vi "Poly_Text_Read.vi"(6 "Auto Increment":bool, 8 "error in":errorcluster, 9 "access (0:read/write)":enum16{"read/write", "read-only", "write-only"}(ring), 10 "operation (0:open)":T1(ring)=enum."open or create", 11 "file path":path) -> (0 "error out":errorcluster, 3 "Text":string)   [LabVIEW 2024, in "Launcher_DTU.lvlib"]
uses:
  Launcher_DTU.lvlib
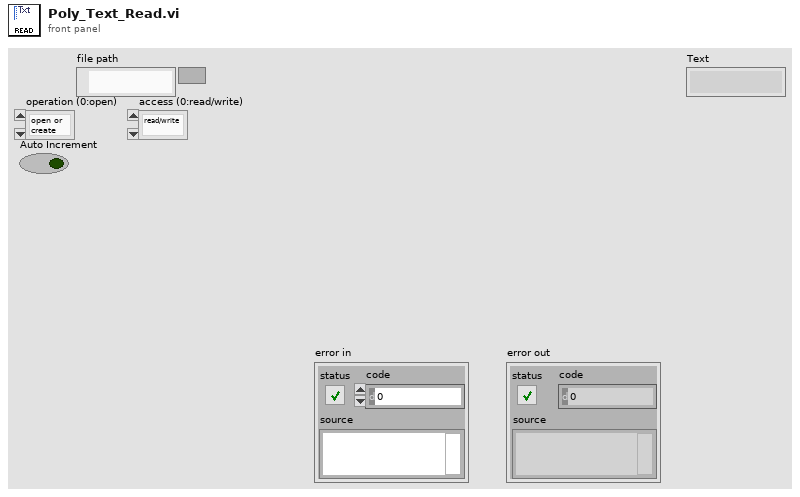
[diagram p1: front panel]
types:
  T1 = enum16{"open", "replace", "create", "open or create", "replace or create", "replace or create with confirmation"}
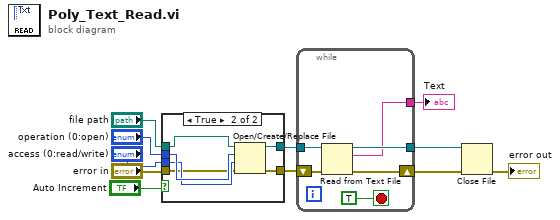
[diagram p0: block diagram]
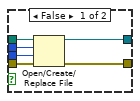
[diagram p2: hidden frame]
diagram:
  n1 = case shown="True" "Auto Increment" {
    tunnel: "error in" -> [w17 w18]
    tunnel: [w16 w23] -> w6
    tunnel: "file path" -> [w15 w22]
    tunnel: "operation (0:open)" -> [w14 w20]
    tunnel: "access (0:read/write)" -> [w13 w19]
    tunnel: [w12 w21] -> w2
    frame False {
      n2 = Open/Create/Replace File(file path (use dialog)=w15, error in=w17, operation (0:open)=w14, access (0:read/write)=w13) -> (refnum out=w12:refnum<file>, error out=w16:errorcluster)  [unwired: 2 in, 1 out]
    }
    frame True {
      n3 = Open/Create/Replace File(file path (use dialog)=w22, error in=w18, operation (0:open)=w20, access (0:read/write)=w19) -> (refnum out=w21:refnum<file>, error out=w23:errorcluster)  [unwired: 2 in, 1 out]
    }
  }
  n4 = while {
    shift-right: [w27] -> w11
    shift-left: w6 -> [w28]
    tunnel: w2 -> [w26]
    tunnel: [w25] -> w9
    tunnel: [w24] -> w8
    stop <- TRUE stop-if-true
    n5 = Read from Text File(file (use dialog)=w26, error in=w28) -> (refnum out=w25:refnum<file>, text=w24:string, error out=w27:errorcluster)  [unwired: 2 in, 1 out]
  }
  "Text" <- w8
  n6 = Close File(refnum=w9, error in=w11) -> (error out=→"error out":errorcluster)  [unwired: 1 out]
